vi "Initialise serial comms.vi"(8 "error in (no error)":errorcluster, 11 "VISA Refnum in":refnum<visa-resource-name>) -> (0 "error out":errorcluster, 2 "Connected?":bool, 3 "VISA Refnum out":refnum<visa-resource-name>)   [LabVIEW 2016]
uses:
  <vilib>/Instr/_visa.llb/VISA Configure Serial Port (Instr).vi
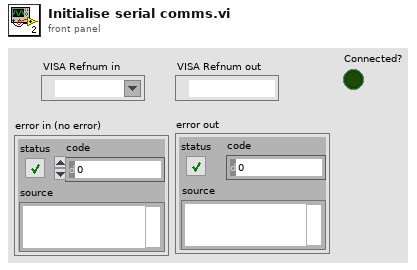
[diagram p1: front panel]
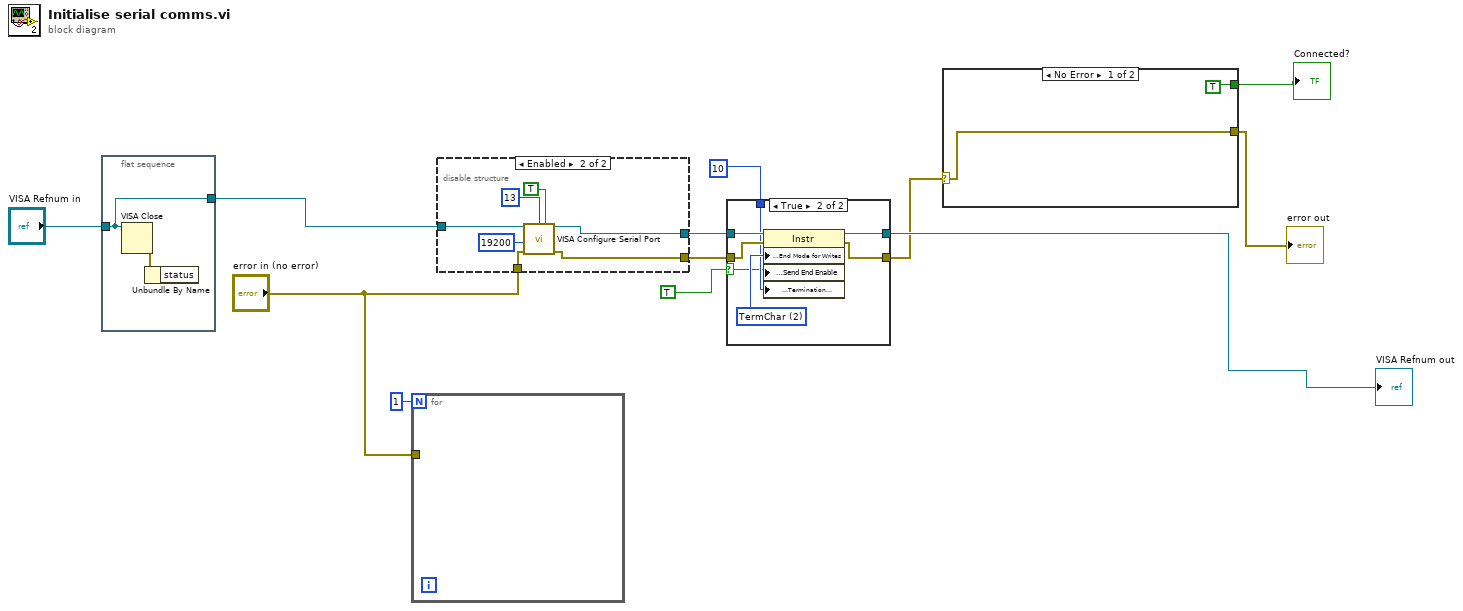
[diagram p0: block diagram]
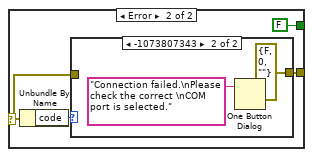
[diagram p2: hidden frame]
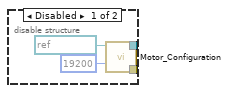
[diagram p5: hidden frame]
diagram:
  n1 = flat-sequence {
    tunnel: "VISA Refnum in" -> [w13]
    tunnel: [w13] -> w1
    frame #0 {
      n2 = VISA Close(VISA resource name=w13) -> (error out=w14:errorcluster)  [unwired: 1 in]
      n3 = Unbundle By Name(w14) -> ()  [unwired: 1 out]
    }
  }
  n4 = for {
    N: 1 -> [_]
    tunnel: "error in (no error)" -> [_]
  }
  n5 = disable-structure shown="Enabled" {
    disable-tunnel: [w16 w24] -> w10
    disable-tunnel: [w15 w23] -> w9
    disable-tunnel: w1 -> [_ w20]
    disable-tunnel: "error in (no error)" -> [_ w19]
    frame Disabled {
      n6 = call "Motor_Configuration.vi"("baud rate"=u32 19200, "VISA resource name"=refnum<visa-resource-name> "COM4") -> ("error out"=w16:errorcluster, "reference out"=w15:refnum<visa-resource-name>)  [unwired: 8 in]
    }
    frame Enabled {
      n7 = call-poly "VISA Configure Serial Port"("VISA resource name"=w20, "termination char\n(0xA = '\\n' = LF)"=u8 13 ("termination char\n(0xA = '\\n' = LF)"), "Enable Termination\nChar (T)"=TRUE ("Enable Termination\nChar (T)"), "baud rate (9600)"=u32 19200, "error in (no error)"=w19) -> ("VISA resource name out"=w23:refnum<visa-resource-name>, "error out"=w24:errorcluster)  [unwired: 5 in, 4 out]
    }
  }
  n8 = case shown="True" TRUE {
    selector: TRUE -> [_ w29]
    tunnel: w9 -> [w26 w34]
    tunnel: w10 -> [w27 w33]
    tunnel: [w26 w32] -> w12
    tunnel: [w27 w28] -> w7
    tunnel: u8 10 ("termination char\n(0xA = '\\n' = LF)") -> [_ w30]
    frame False {
    }
    frame True {
      w31 = u16 2 items=["None", "LastBit", "TermChar", "Break"] ("Serial Settings:Serial End Mode for Writes")
      n9 = property class="Instr"(reference=w34, error in=w33, "Serial Settings:End Mode for Writes"=w31, "Message Based Settings:Send End Enable"=w29, "Message Based Settings:Termination Character"=w30) -> (reference out=w32:refnum<visa-resource-name>, error out=w28:errorcluster)
    }
  }
  "VISA Refnum out" <- w12
  n10 = case shown="No Error" w7 {
    selector: w7 -> [w36 w39]
    tunnel: [w36 w38] -> w6
    tunnel: [TRUE FALSE] -> w5
    frame No Error {
    }
    frame Error {
      n11 = Unbundle By Name(w39) -> ("code"=w40:i32)
      n12 = case shown="-1073807343" w40 {
        tunnel: w39 -> [w41 _]
        tunnel: [w41 errorcluster {"status"=FALSE, "code"=0, "source"=""} ("error IO")] -> w38
        frame 0, Default {
        }
        frame -1073807343 {
          n13 = One Button Dialog(message="Connection failed.\nPlease check the correct \nCOM port is selected.") -> ()  [unwired: 1 in, 1 out]
        }
      }
    }
  }
  "error out" <- w6
  "Connected?" <- w5
